vi "New JSON Array (String).vi"(8 "error in (no error)":errorcluster, 10 "String Array":string[](array[string])) -> (0 "error out":errorcluster, 3 "JSON Array out":refnum<class "JSON Array.lvclass">)   [LabVIEW 2016, in "LVJSON.lvlib" / "JSON Array.lvclass"]
doc: "Creates a new JSON Array initialized with JSON Boolean objects of the values specified by String Array"
uses:
  JSON Array.lvclass
  JSON String/JSON String.lvclass
  C:/Users/tblair/Documents/Git Projects/JSON-Support-for-LabVIEW/Source/JSON Data Classes/JSON Datatype/JSON Null.lvclass
  JSON String/New JSON String.vi
  JSON Helper/JSON Helper.lvclass
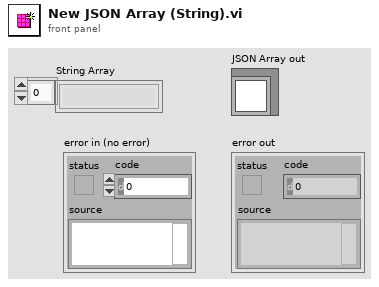
[diagram p1: front panel]
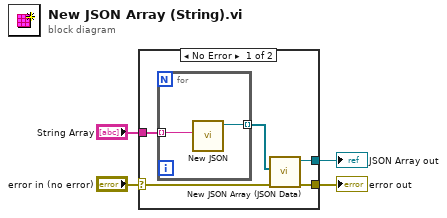
[diagram p0: block diagram]
diagram:
  n1 = case shown="No Error" "error in (no error)" {
    selector: "error in (no error)" -> [w6 w12]
    tunnel: [w5 w12] -> w3
    tunnel: [w8 _] -> w2
    tunnel: "String Array" -> [w9 _]
    frame No Error {
      n2 = for {
        tunnel: w9 -> [w11] mode=indexing
        tunnel: [w10] -> w7 mode=indexing
        n3 = call-poly "New JSON.vi"("value"=w11) -> ("JSON String out"=w10:refnum<class "JSON String.lvclass">)  [unwired: 9 in, 1 out]
      }
      n4 = call "New JSON Array (JSON Data).vi"("error in (no error)"=w6, "JSON Datatypes"=w7) -> ("error out"=w5:errorcluster, "JSON Array out"=w8:refnum<class "JSON Array.lvclass">)  [unwired: 8 in]
    }
    frame Error {
    }
  }
  "error out" <- w3
  "JSON Array out" <- w2
